vi "LWXPS_EventAdd.vi"(0 "Event Name":string, 1 "Positioner Name":string, 2 "XPS Reference IN":refnum<k24>, 5 "Event Parameter":string, 7 "Action Name":string, 9 "Action Parameter 1":string, 11 "Action Parameter 2":string, 12 "Action Parameter 3":string, 13 "LabVIEW error IN":errorcluster) -> (4 "XPS Reference OUT":refnum<k24>, 6 "Returned error code":i32, 8 "XPS Error String":string, 15 "LabVIEW error OUT":errorcluster)   [LabVIEW 2014]
uses:
  D:/XPSQ8_LabView_Library/Development/Source/Dll/Newport.XPS.CommandInterface.dll
  Dll/Newport.XPS.CommandInterface.dll
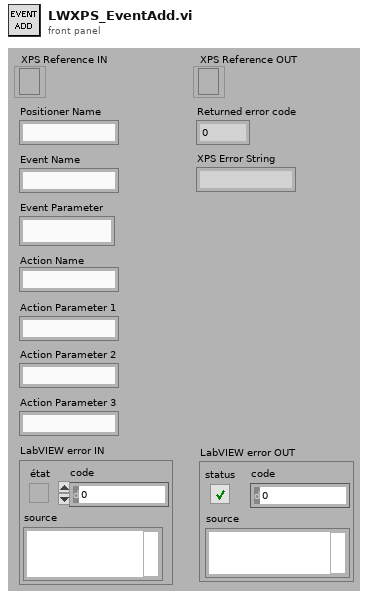
[diagram p1: front panel]
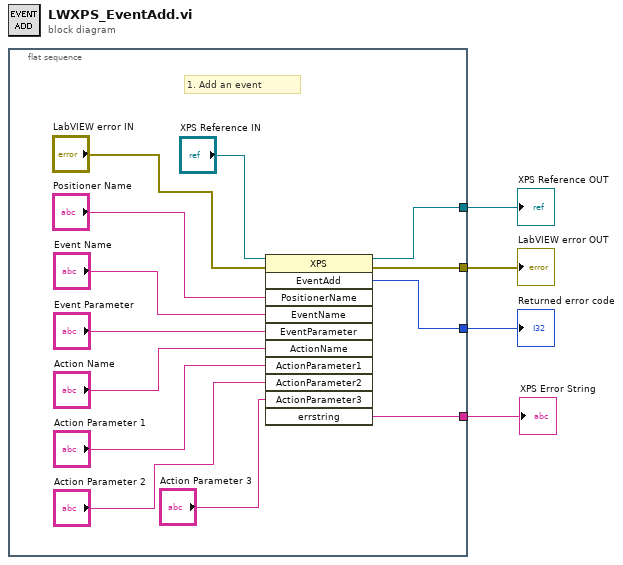
[diagram p0: block diagram]
diagram:
  n1 = flat-sequence {
    tunnel: [w15] -> w4
    tunnel: [w17] -> w3
    tunnel: [w14] -> w1
    tunnel: [w13] -> w2
    frame #0 {
      # "1. Add an event"
      n2 = invoke class="XPS" method="EventAdd"(reference="XPS Reference IN", error in="LabVIEW error IN", "PositionerName"="Positioner Name", "EventName"="Event Name", "EventParameter"="Event Parameter", "ActionName"="Action Name", "ActionParameter1"="Action Parameter 1", "ActionParameter2"="Action Parameter 2", "ActionParameter3"="Action Parameter 3") -> (reference out=w15:refnum<k24>, error out=w17:errorcluster, "EventAdd"=w14:i32, "errstring"=w13:string)  [unwired: 2 in, 7 out]
    }
  }
  "XPS Reference OUT" <- w4
  "LabVIEW error OUT" <- w3
  "XPS Error String" <- w2
  "Returned error code" <- w1
